vi "Debug UI.vi"(11 "Terminal in":refnum<class "Terminal.lvclass">) -> ()   [LabVIEW 2020, in "Terminal.lvlib" / "Terminal.lvclass"]
uses:
  Terminal.lvclass
  Parse State.ctl
  Buffer State.ctl
  Cursor.ctl
  Position.ctl
  Text Attributes.ctl
  Buffer.ctl
  Terminal Options.ctl
  Color Scheme.ctl
  Color.ctl
  Font Metrics.ctl
  Terminal.lvclass/Terminal.ctl
  <vilib>/IlluminatedG/lv-stream/Connection/Connection.lvclass
  TermBuffer/TermBuffer.lvclass
  Terminal.lvlib
panel:
  out "Touched Lines":cluster{"Touched Lines":bool[]}[](array[cluster])
  out "Buffer Status":T1(array[cluster])
  out "User Input Enabled":bool
  out "Pause Read Loop":bool
  out "Buffer":T2
  out "Close Read Loop":bool
  out "Scroll":i32
  out "Font Metrics":T3
  out "Terminal Options":T4={"Implied CR with LF"=TRUE, "Local Echo"=FALSE, "Tab Width"=8, "Color Scheme"={"Black"=2302755, "Red"=16711695, "Green"=9232651, "Yellow"=16759040, "Blue"=36344, "Magenta"=7160742, "Cyan"=55531, "White"=15132390, "Bright Black"=4473924, "Bright Red"=16721728, "Bright Green"=11264347, "Bright Yellow"=16765506, "Bright Blue"=37631, "Bright Magenta"=10117099, "Bright Cyan"=6815728, "Bright White"=16777215}, "Default FG"=37, "Default BG"=90, "History Length"=5000, "Font Face"="Fixedsys", "Font Size"=14, "Rows"=24, "Cols"=80} {"Default BG" items=["Black"=30, "Red"=31, "Green"=32, "Yellow"=33, "Blue"=34, "Magenta"=35, "Cyan"=36, "White"=37, "Gray"=90, "Bright Red"=91, "Bright Green"=92, "Bright Yellow"=93, "Bright Blue"=94, "Bright Magenta"=95, "Bright Cyan"=96, "Bright White"=97]; "Default FG" items=["Black"=30, "Red"=31, "Green"=32, "Yellow"=33, "Blue"=34, "Magenta"=35, "Cyan"=36, "White"=37, "Gray"=90, "Bright Red"=91, "Bright Green"=92, "Bright Yellow"=93, "Bright Blue"=94, "Bright Magenta"=95, "Bright Cyan"=96, "Bright White"=97]}
  out "Parse State":T7
  out "Read Loop Running":bool
  out "Connected":bool
  out "Connection Class":string
  # "Scrollback"
  # "Primary"
  # "Alternate"
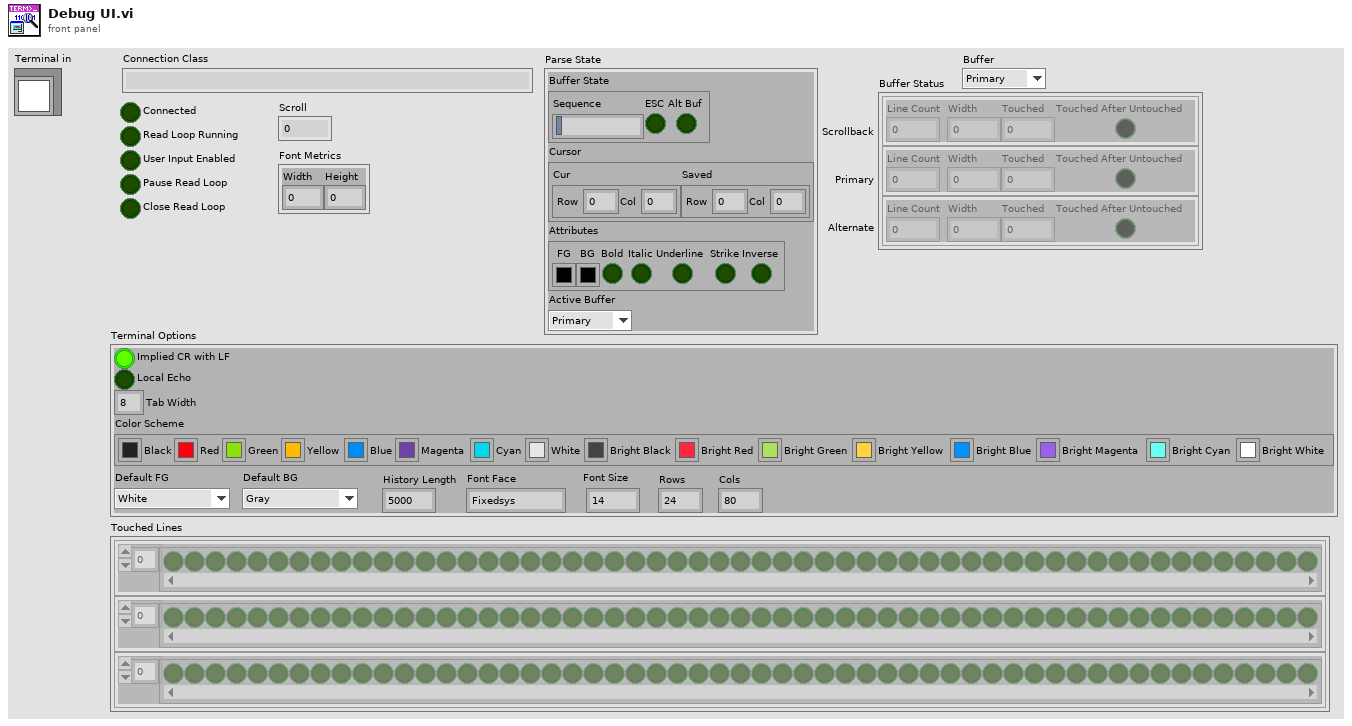
[diagram p1: front panel]
types:
  T1 = cluster{"Line Count":i32, "Width":i32, "Touched":i32, "Touched After Untouched":bool}[]
  T2 = typedef "Terminal.lvlib/Buffer.ctl" = enum16{"Primary", "Alternate"}
  T3 = typedef "Terminal.lvlib/Terminal.lvclass/Font Metrics.ctl" = cluster{"Width":i16, "Height":i16}
  T4 = typedef "Terminal.lvlib/Terminal Options.ctl" = cluster{"Implied CR with LF":bool, "Local Echo":bool, "Tab Width":i32, "Color Scheme":T5, "Default FG":T6, "Default BG":T6, "History Length":i32, "Font Face":string, "Font Size":i16, "Rows":i32, "Cols":i32}
  T5 = typedef "Terminal.lvlib/Color Scheme.ctl" = cluster{"Black":u32, "Red":u32, "Green":u32, "Yellow":u32, "Blue":u32, "Magenta":u32, "Cyan":u32, "White":u32, "Bright Black":u32, "Bright Red":u32, "Bright Green":u32, "Bright Yellow":u32, "Bright Blue":u32, "Bright Magenta":u32, "Bright Cyan":u32, "Bright White":u32}
  T6 = typedef "Terminal.lvlib/Color.ctl" = i8
  T7 = typedef "Terminal.lvlib/Terminal.lvclass/Parse State.ctl" = cluster{"Buffer State":T8, "Cursor":T9, "Attributes":T11, "Active Buffer":T2}
  T8 = typedef "Terminal.lvlib/Terminal.lvclass/Buffer State.ctl" = cluster{"Sequence":string, "ESC":bool, "Alt Buf":bool}
  T9 = typedef "Terminal.lvlib/Terminal.lvclass/Cursor.ctl" = cluster{"Cur":T10, "Saved":T10}
  T10 = typedef "Terminal.lvlib/Terminal.lvclass/Position.ctl" = cluster{"Row":i32, "Col":i32}
  T11 = typedef "Terminal.lvlib/Text Attributes.ctl" = cluster{"FG":u32, "BG":u32, "Bold":bool, "Italic":bool, "Underline":bool, "Strike":bool, "Inverse":bool}
  T12 = typedef "Terminal.lvlib/Terminal.lvclass/Ref Data.ctl" = cluster{"Connection":refnum<class "Connection.lvclass">, "Read Loop Running":bool, "Parse State":T7, "Terminal Options":T4, "Font Metrics":T3, "Scroll":i32, "Close Read Loop":bool, "Buffer":T2, "Pause Read Loop":bool, "User Input Enabled":bool}
  T13 = cluster{"Line Count":i32, "Width":i32, "index of element":i32, bool}
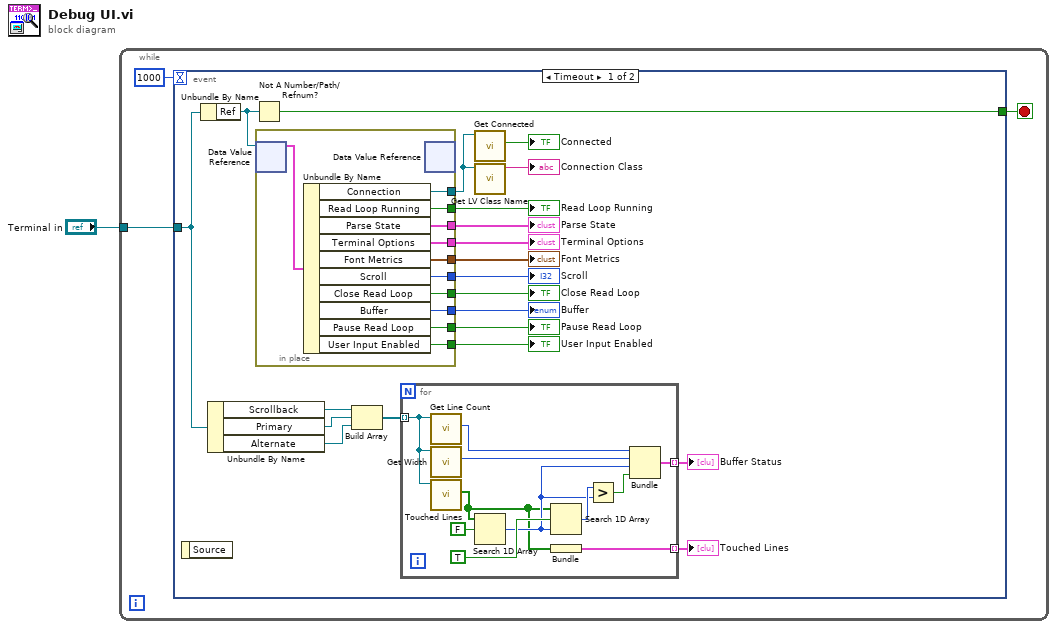
[diagram p0: block diagram]
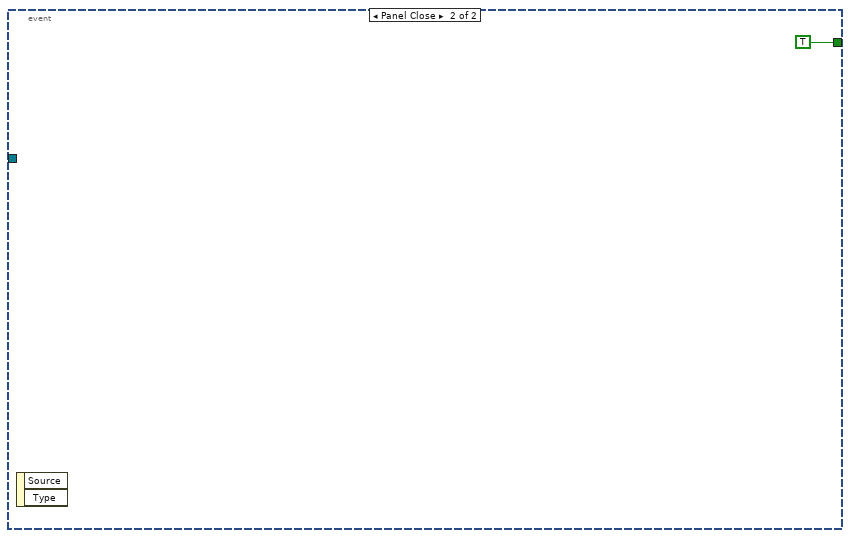
[diagram p2: hidden frame]
diagram:
  n1 = while {
    tunnel: "Terminal in" -> [w3]
    stop <- w2 stop-if-true
    n2 = event shown="[0] Timeout" {
      selector: _ -> [_ _]
      dyn-events: _ -> [_ _]
      timeout: 1000 -> [_ _]
      tunnel: w3 -> [w11 _]
      tunnel: [w25 TRUE] -> w2
      event Timeout {
        n3 = event-data() -> ()  [unwired: 1 in, 1 out]
        n4 = Unbundle By Name(w11) -> ("Ref"=w24:refnum<data-value>)
        n5 = Unbundle By Name(w11) -> ("Scrollback"=w10:refnum<class "TermBuffer.lvclass">, "Primary"=w9:refnum<class "TermBuffer.lvclass">, "Alternate"=w8:refnum<class "TermBuffer.lvclass">)
        n6 = Not A Number/Path/Refnum?(number/path/refnum=w24) -> (NaN/Path/Refnum?=w25:bool)
        n7 = in-place {
          in-place-border: [w46] -> w23
          in-place-border: [w45] -> w20
          in-place-border: [w44] -> w19
          in-place-border: [w43] -> w18
          in-place-border: [w42] -> w17
          in-place-border: [w41] -> w16
          in-place-border: [w40] -> w15
          in-place-border: [w39] -> w14
          in-place-border: [w38] -> w13
          in-place-border: [w37] -> w12
          n8 = in-place-dvr #1(w24) -> (w47:T12)  [unwired: 1 out]
          n9 = Unbundle By Name(w47) -> ("Connection"=w46:refnum<class "Connection.lvclass">, "Read Loop Running"=w45:bool, "Parse State"=w44:T7, "Terminal Options"=w43:T4, "Font Metrics"=w42:T3, "Scroll"=w41:i32, "Close Read Loop"=w40:bool, "Buffer"=w39:T2, "Pause Read Loop"=w38:bool, "User Input Enabled"=w37:bool)
          n10 = in-place-dvr #1() -> ()  [unwired: 1 in, 2 out]
        }
        "Read Loop Running" <- w20
        "Parse State" <- w19
        "Terminal Options" <- w18
        "Font Metrics" <- w17
        "Scroll" <- w16
        "Close Read Loop" <- w15
        "Buffer" <- w14
        "Pause Read Loop" <- w13
        "User Input Enabled" <- w12
        n11 = Build Array(w10, w9, w8) -> (w7:refnum<class "TermBuffer.lvclass">[])
        n12 = for {
          tunnel: w7 -> [w36] mode=indexing
          tunnel: [w28] -> w6 mode=indexing
          tunnel: [w26] -> w5 mode=indexing
          n13 = call "Get Line Count.vi"("TermBuffer in"=w36) -> ("Line Count"=w32:i32)  [unwired: 8 in, 2 out]
          n14 = call "Get Width.vi"("TermBuffer in"=w36) -> ("Width"=w31:i32)  [unwired: 8 in, 2 out]
          n15 = call "Touched Lines.vi"("TermBuffer in"=w36) -> ("Touched Lines"=w27:bool[])  [unwired: 8 in, 2 out]
          n16 = Search 1D Array(1D array=w27, element=FALSE) -> (index of element=w30:i32)  [unwired: 1 in]
          n17 = Search 1D Array(1D array=w27, element=TRUE, start index (0)=w30) -> (index of element=w33:i32)
          n18 = Bundle("Touched Lines"=w27) -> (w26:cluster{"Touched Lines":bool[]})  [unwired: 1 in]
          n19 = Greater?(x=w33, y=w30) -> (0:w29:bool)
          n20 = Bundle("Line Count"=w32, "Width"=w31, "index of element"=w30, w29) -> (w28:T13)  [unwired: 1 in]
        }
        "Buffer Status" <- w6
        "Touched Lines" <- w5
        n21 = call <vilib>:"Get Connected.vi"("Connection in"=w23) -> ("Connected"=→"Connected":bool)  [unwired: 8 in, 2 out]
        n22 = call <vilib>:"Get LV Class Name.vi"("object"=w23) -> ("class name"=→"Connection Class":string)  [unwired: 9 in, 1 out]
      }
      event Panel Close {
        n23 = event-data() -> ()  [unwired: 1 in, 2 out]
      }
    }
  }
